vi "tiff stack write module.vi"(2 "Compression Type (None)":i32(ring) items=["None", "JPEG", "Run Length Encoded", "Zip"], 4 "Convert to U16?":bool, 5 "action":enum16{"open", "save", "close"}(ring)=enum."close", 6 "Add metadata? (T)":bool=TRUE, 8 "error in":errorcluster, 9 "file Path":path=path "C:/Users/BoasLab/Documents/Data/Alazar data/B-line/data/test.tif", 10 "Image (U8, U16, I16)":T1, 11 "ImageDescription":string) -> (0 "error out":errorcluster)   [LabVIEW 2018]
uses:
  <vilib>/vision/Image Controls.llb/IMAQ Image.ctl
  Dans Tiff Stack Code/File IO/Image/Tiff/Tiff reader.lvlib
  <vilib>/vision/NI_Vision_Development_Module.lvlib
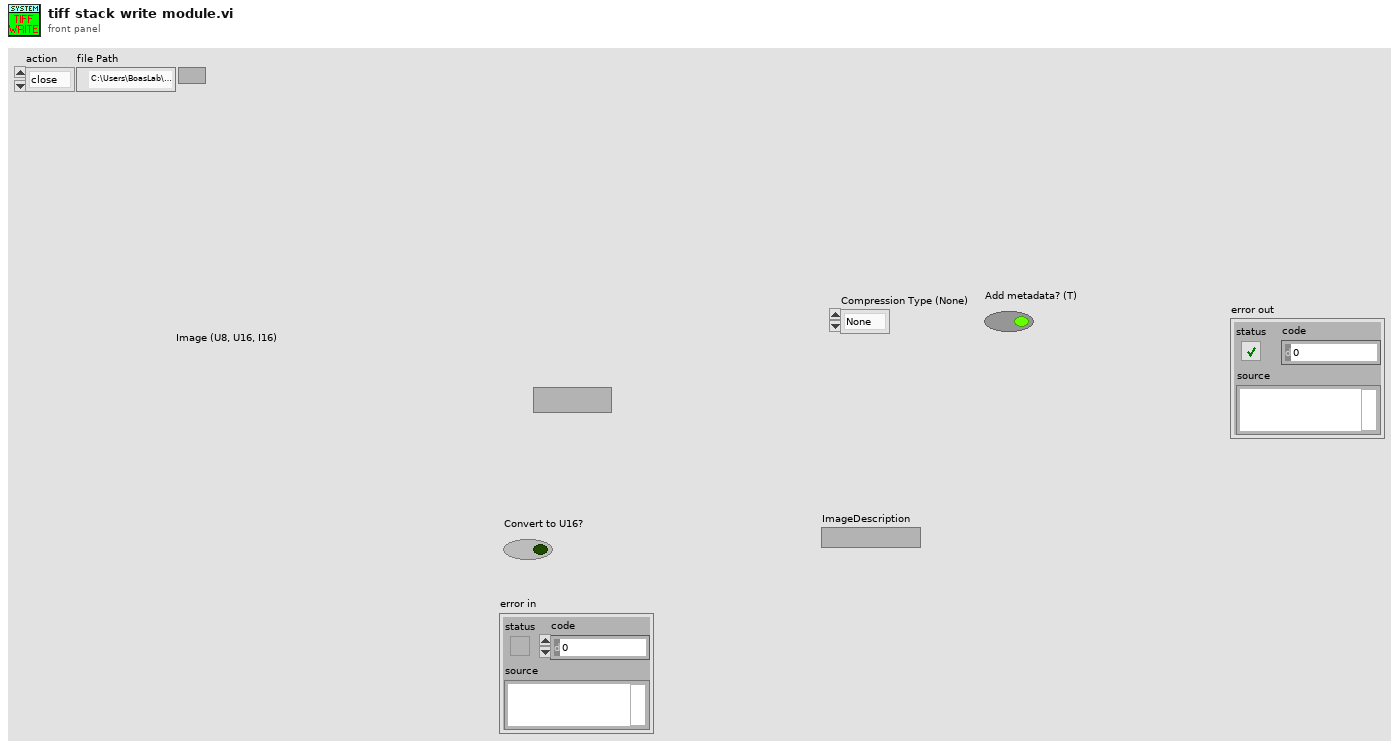
[diagram p1: front panel]
types:
  T1 = typedef "IMAQ Image.ctl" = refnum<image>
  T2 = cluster{"Rows Per Strip":i32, "Photometric":i32, "Compression Type":i32}
  T3 = enum16{"open", "replace", "create", "open or create", "replace or create", "replace or create with confirmation"}
  T4 = typedef "Image Type" = u32
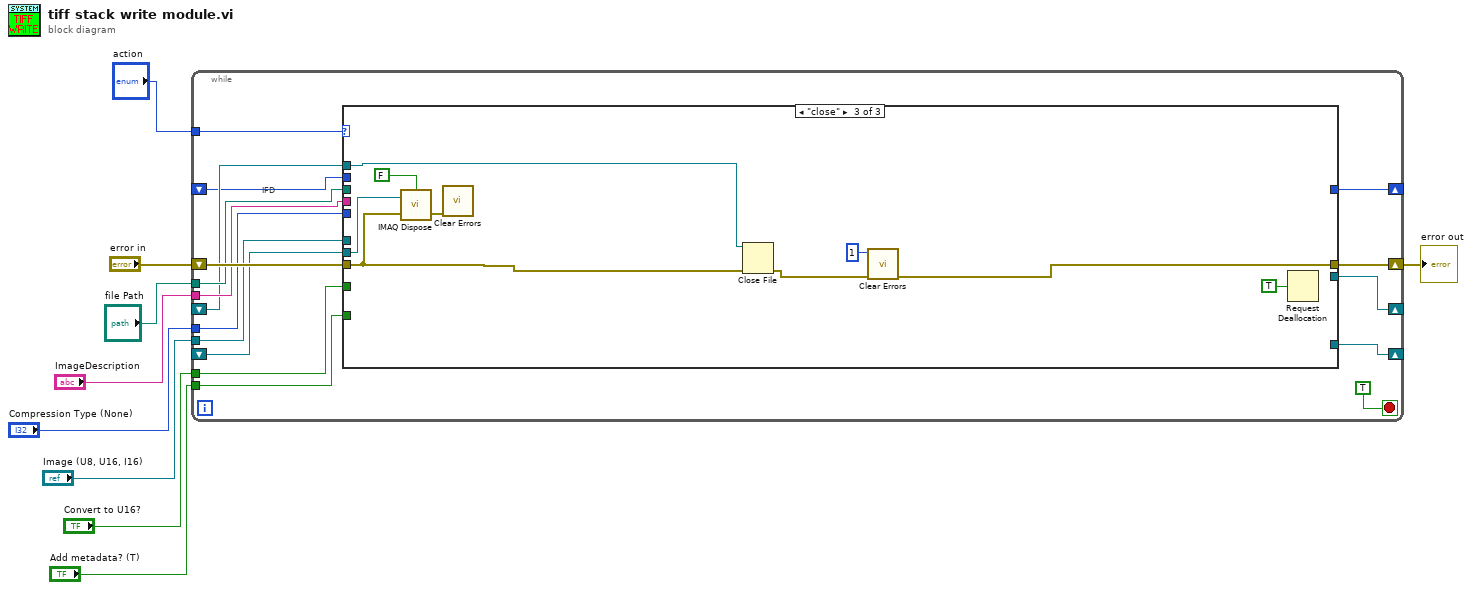
[diagram p0: block diagram]
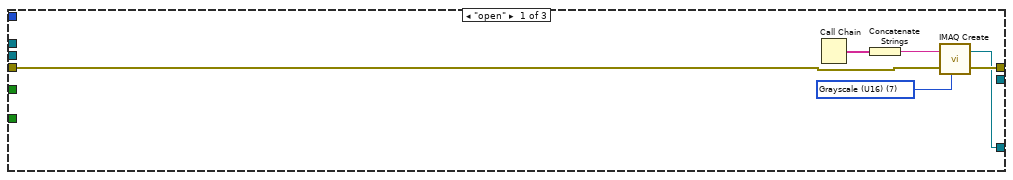
[diagram p2: hidden frame]
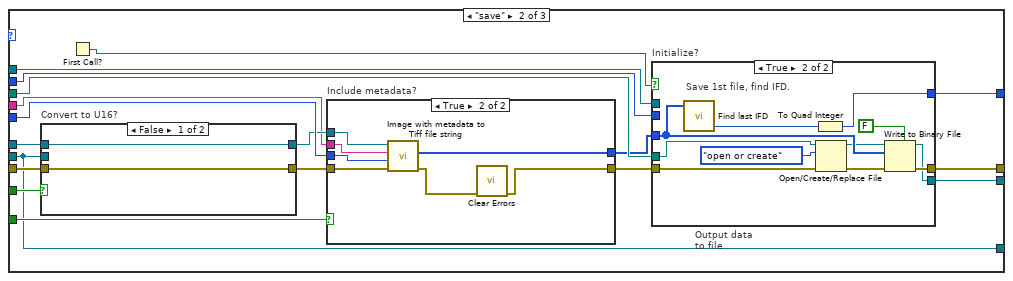
[diagram p3: hidden frame]
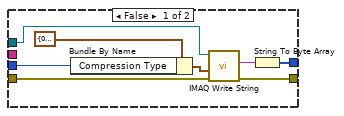
[diagram p4: hidden frame]
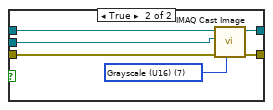
[diagram p5: hidden frame]
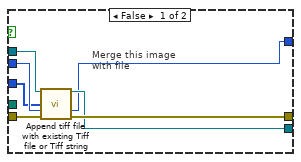
[diagram p6: hidden frame]
diagram:
  n1 = while {
    tunnel: "Image (U8, U16, I16)" -> [w20]
    tunnel: "Add metadata? (T)" -> [w17]
    tunnel: "file Path" -> [w18]
    tunnel: "ImageDescription" -> [w19]
    tunnel: "Convert to U16?" -> [w16]
    tunnel: "Compression Type (None)" -> [w15]
    tunnel: "action" -> [w25]
    shift-right: [w24] -> w2
    shift-left: "error in" -> [w23]
    shift-right: [w22] -> _
    shift-left: _ -> [w21]
    shift-right: [w14] -> _
    shift-left: _ -> [w13]
    shift-right: [w11] -> _
    shift-left: _ -> [w10]
    stop <- TRUE stop-if-true
    # "IFD"
    n2 = case shown="\"close\"" w25 {
      tunnel: [w28 w42 w92] -> w24
      tunnel: w23 -> [w26 w46 w95]
      tunnel: [w27 w41 _] -> w22
      tunnel: w21 -> [_ w41 w96]
      tunnel: w20 -> [_ w49 _]
      tunnel: w19 -> [_ w33 _]
      tunnel: w18 -> [_ w48 _]
      tunnel: w17 -> [_ w47 _]
      tunnel: w16 -> [_ w45 _]
      tunnel: w15 -> [_ w44 _]
      tunnel: [_ w43 _] -> w14
      tunnel: w13 -> [_ w34 w94]
      tunnel: [_ w40 _] -> w11
      tunnel: w10 -> [_ w39 _]
      frame "open" {
        w31 = T4 7 items=["Grayscale (U8)", "Grayscale (I16)", "Grayscale (SGL)", "Complex (CSG)", "RGB (U32)", "HSL (U32)", "RGB (U64)", "Grayscale (U16)"] ("Image Type")
        n3 = Call Chain() -> (call chain=w30:string[])
        n4 = Concatenate Strings(w30) -> (w29:string)
        n5 = call "IMAQ Create"("Image Name"=w29, "Image Type"=w31, "error in (no error)"=w26) -> ("New Image"=w27:T1, "error out"=w28:errorcluster)  [unwired: 1 in, 1 out]
      }
      frame "save" {
        # "Output data\nto file"
        n6 = case "Convert to U16?" shown="False" w45 {
          tunnel: w46 -> [w65 w72]
          tunnel: [w65 w71] -> w37
          tunnel: w49 -> [w66 w70]
          tunnel: w41 -> [_ w69]
          tunnel: [w66 w67] -> w38
          frame False {
          }
          frame True {
            w68 = T4 7 items=["Grayscale (U8)", "Grayscale (I16)", "Grayscale (SGL)", "Complex (CSG)", "RGB (U32)", "HSL (U32)", "RGB (U64)", "Grayscale (U16)"] ("Image Type")
            n7 = call "IMAQ Cast Image"("Image Type"=w68, "error in (no error)"=w72, "Image Dst"=w69, "Image Src"=w70) -> ("error out"=w71:errorcluster, "Image Dst Out"=w67:T1)  [unwired: 2 in, 4 out]
          }
        }
        n8 = First Call?() -> (First Call?: T/F=w32:bool)
        n9 = case "Include metadata?" shown="True" w47 {
          tunnel: w38 -> [w52 w64]
          tunnel: w37 -> [w53 w63]
          tunnel: [w54 w58] -> w36
          tunnel: [w50 w62] -> w35
          tunnel: w44 -> [w51 w61]
          tunnel: w33 -> [_ w60]
          frame False {
            n10 = Bundle By Name(cluster=T2 {"Rows Per Strip"=0, "Photometric"=1, "Compression Type"=0} ("TIFF Options"), "Compression Type"=w51) -> (w56:T2)
            n11 = call-poly "IMAQ Write String"("error in (no error)"=w53, "TIFF Options"=w56, "Image"=w52) -> ("error out"=w54:errorcluster, "FileString"=w55:string)  [unwired: 2 in, 5 out]
            n12 = String To Byte Array(string=w55) -> (unsigned byte array=w50:u8[])
          }
          frame True {
            n13 = call "Image with metadata to Tiff file string.vi"("error in"=w63, "Compression Type (None)"=w61, "ImageDescription string\n(must be at least 5 char long)"=w60, "img"=w64) -> ("error out"=w59:errorcluster, "Tiff file out (unsigned byte array)"=w62:u8[])  [unwired: 2 out]
            n14 = call <vilib>:"Clear Errors.vi"("error in (no error)"=w59) -> ("error out"=w58:errorcluster)  [unwired: 5 in, 1 out]
          }
        }
        n15 = case "Initialize?" shown="True" w32 {
          tunnel: w36 -> [w78 w82]
          tunnel: w48 -> [_ w84]
          tunnel: [w79 w90] -> w42
          tunnel: [w77 w89] -> w43
          tunnel: w39 -> [w76 _]
          tunnel: [w75 w86] -> w40
          tunnel: w35 -> [w74 w85]
          tunnel: w34 -> [w73 _]
          frame False {
            # "Merge this image\nwith file"
            n16 = call "Append tiff file with existing Tiff file or Tiff string.vi"("Existing Tiff File (A) refnum"=w73, "Tiff file (B)\n (unsigned byte array)"=w74, "Location in existing file of\nit's last page's \n\"next IFD pointer\""=w76, "error in"=w78) -> ("File refnum out"=w77:refnum<file>, "Location in new file of\nit's last page's \n\"next IFD pointer\""=w75:i64, "error out"=w79:errorcluster)  [unwired: 3 in, 6 out]
          }
          frame True {
            # "Save 1st file, find IFD."
            n17 = call "Find last IFD.vi"("TIFF Data in"=w85) -> ("Location in byte stream of last IFD pointer.  This\nis the word to change if you are adding another page\nto the file."=w87:i32)  [unwired: 4 out]
            n18 = To Quad Integer(1:w87) -> (0:w86:i64)
            n19 = Open/Create/Replace File(file path (use dialog)=w84, error in=w82, operation (0:open)=T3."open or create") -> (refnum out=w80:refnum<file>, error out=w81:errorcluster)  [unwired: 3 in, 1 out]
            n20 = Write to Binary File(file (use dialog)=w80, data=w85, error in=w81, 5:FALSE ("prepend array or string size? (T)")) -> (refnum out=w89:refnum<file>, error out=w90:errorcluster)  [unwired: 1 in, 2 out]
          }
        }
      }
      frame "close" {
        n21 = call "IMAQ Dispose"("All Images? (No)"=FALSE, "Image"=w96, "error in (no error)"=w95) -> ("error out"=w99:errorcluster)  [unwired: 3 out]
        n22 = call <vilib>:"Clear Errors.vi"("error in (no error)"=w99) -> ()  [unwired: 1 in, 6 out]
        n23 = Close File(refnum=w94, error in=w95) -> (error out=w93:errorcluster)  [unwired: 1 out]
        n24 = call <vilib>:"Clear Errors.vi"("error in (no error)"=w93, "specific error code to clear (0: all)"=1) -> ("error out"=w92:errorcluster)  [unwired: 4 in, 1 out]
        n25 = Request Deallocation(TRUE ("flag")) -> ()
      }
    }
  }
  "error out" <- w2
